vi "Read Video.vi"(8 "error in (no error)":errorcluster, 11 "input cluster":T4={"Video Resolution"=enum."FREENECT_RESOLUTION_LOW", "Video Format"=enum."FREENECT_VIDEO_RGB", "Depth Format"=enum."FREENECT_DEPTH_11BIT", "Depth Resolution"=enum."FREENECT_RESOLUTION_LOW"}) -> (0 "error out":errorcluster, 1 "raw data":u16[](array[numeric]), 3 "RGB image":picture)   [LabVIEW 2015]
uses:
  Video Resolution Control.ctl
  Video Format Control.ctl
  Depth Resolution Control.ctl
  <vilib>/picture/picture.llb/Draw True-Color Pixmap.vi
  libkinect_wrapper.dll
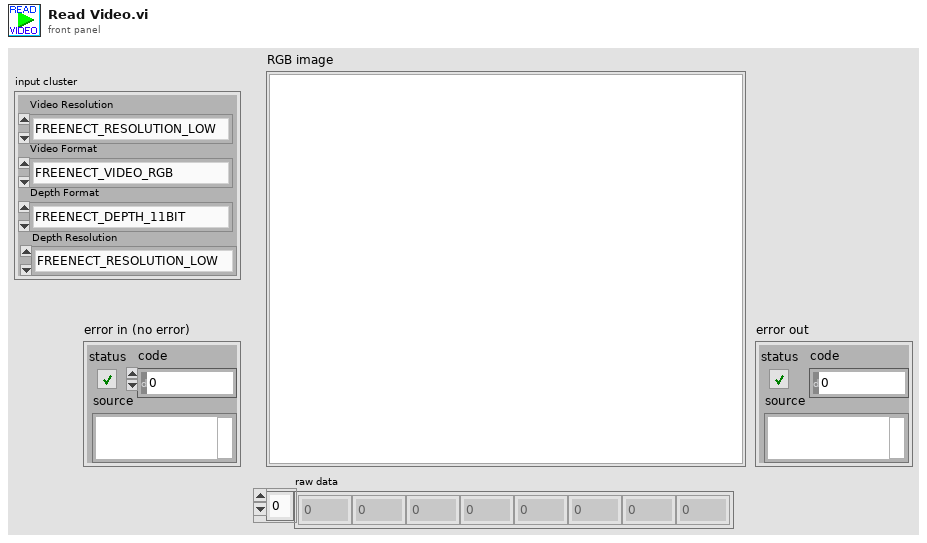
[diagram p1: front panel]
types:
  T1 = typedef "Video Resolution Control.ctl" = enum32{"FREENECT_RESOLUTION_LOW", "FREENECT_RESOLUTION_MEDIUM", "FREENECT_RESOLUTION_HIGH"}
  T2 = typedef "Video Format Control.ctl" = enum32{"FREENECT_VIDEO_RGB", "FREENECT_VIDEO_BAYER", "FREENECT_VIDEO_IR_8BIT", "FREENECT_VIDEO_IR_10BIT", "FREENECT_VIDEO_IR_10BIT_PACKED", "FREENECT_VIDEO_YUV_RGB", "FREENECT_VIDEO_YUV_RAW"}
  T3 = typedef "Depth Resolution Control.ctl" = enum16{"FREENECT_RESOLUTION_TINY", "FREENECT_RESOLUTION_LOW", "FREENECT_RESOLUTION_MEDIUM"}
  T4 = cluster{"Video Resolution":T1, "Video Format":T2, "Depth Format":enum32{"FREENECT_DEPTH_11BIT", "FREENECT_DEPTH_10BIT", "FREENECT_DEPTH_11BIT_PACKED", "FREENECT_DEPTH_10BIT_PACKED", "FREENECT_DEPTH_REGISTERED", "FREENECT_DEPTH_MM"}, "Depth Resolution":T3}
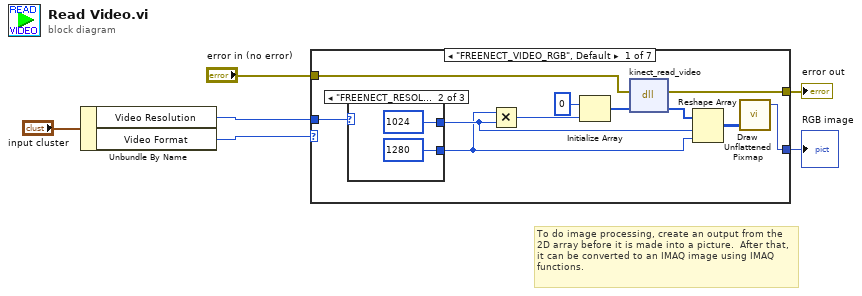
[diagram p0: block diagram]
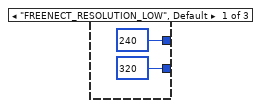
[diagram p2: hidden frame]
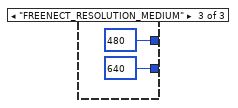
[diagram p3: hidden frame]
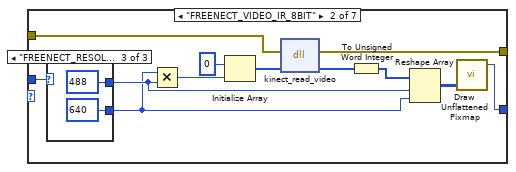
[diagram p4: hidden frame]
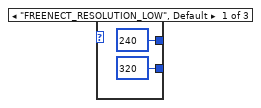
[diagram p5: hidden frame]
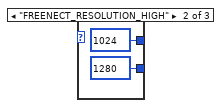
[diagram p6: hidden frame]
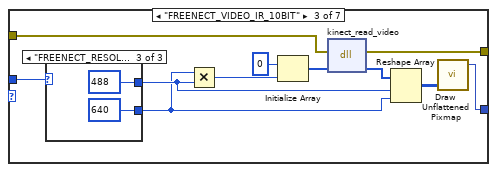
[diagram p7: hidden frame]
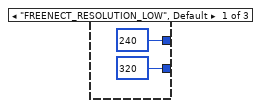
[diagram p8: hidden frame]
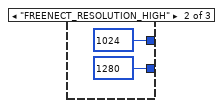
[diagram p9: hidden frame]
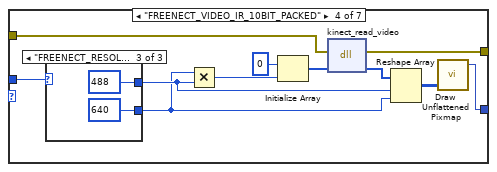
[diagram p10: hidden frame]
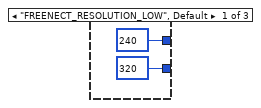
[diagram p11: hidden frame]
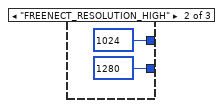
[diagram p12: hidden frame]
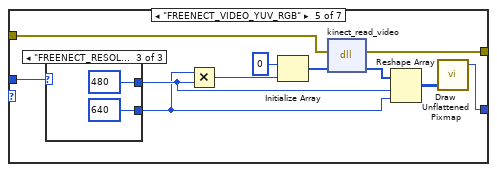
[diagram p13: hidden frame]
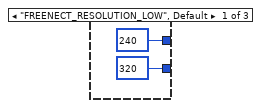
[diagram p14: hidden frame]
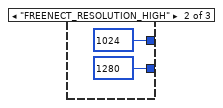
[diagram p15: hidden frame]
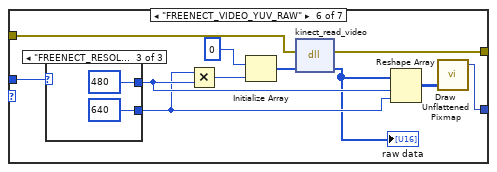
[diagram p16: hidden frame]
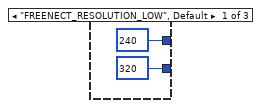
[diagram p17: hidden frame]
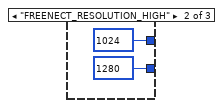
[diagram p18: hidden frame]
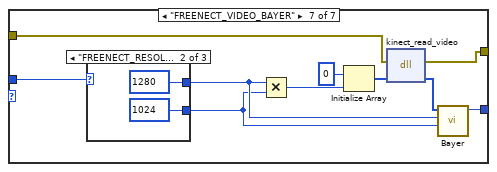
[diagram p19: hidden frame]
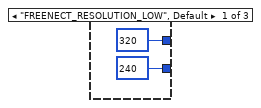
[diagram p20: hidden frame]
diagram:
  # "To do image processing, create an output from the 2D array before it is made into a picture.  After that, it can be converted to an IMAQ image using IMAQ functions."
  n1 = Unbundle By Name("input cluster") -> ("Video Resolution"=w4:T1, "Video Format"=w5:T2)
  n2 = case shown="\"FREENECT_VIDEO_RGB\", Default" w5 {
    tunnel: w4 -> [w17 w27 w42 w61 w86 w103 w112]
    tunnel: [w11 w29 w44 w63 w80 w94 w113] -> w3
    tunnel: "error in (no error)" -> [w10 w28 w43 w62 w79 w99 w115]
    tunnel: [w9 w30 w45 w64 w78 w98 w114] -> w1
    frame "FREENECT_VIDEO_RGB", Default {
      n3 = case shown="\"FREENECT_RESOLUTION_HIGH\"" w17 {
        tunnel: [240 1024 480] -> w8
        tunnel: [320 1280 640] -> w7
        frame "FREENECT_RESOLUTION_LOW", Default {
        }
        frame "FREENECT_RESOLUTION_HIGH" {
        }
        frame "FREENECT_RESOLUTION_MEDIUM" {
        }
      }
      n4 = Multiply(x=w7, y=w8) -> (x*y=w16:i32)
      n5 = Initialize Array(u32 0 ("U32"), w16) -> (w15:u32[])
      n6 = dll-call lib="libkinect_wrapper.*" fn="kinect_read_video"(error in=w10, "video"=w15) -> (error out=w9:errorcluster, "video"=w13:u32[])  [unwired: 3 in, 1 out]
      n7 = Reshape Array(w13, w8, w7) -> (w12:u32[][])
      n8 = call-poly <vilib>:"Draw Unflattened Pixmap.vi"("data (RGB format)"=w12) -> ("new picture"=w11:picture)  [unwired: 8 in]
    }
    frame "FREENECT_VIDEO_IR_8BIT" {
      n9 = case shown="\"FREENECT_RESOLUTION_MEDIUM\"" w27 {
        tunnel: [240 1024 488] -> w32
        tunnel: [320 1280 640] -> w31
        frame "FREENECT_RESOLUTION_LOW", Default {
        }
        frame "FREENECT_RESOLUTION_HIGH" {
        }
        frame "FREENECT_RESOLUTION_MEDIUM" {
        }
      }
      n10 = Multiply(x=w31, y=w32) -> (x*y=w35:i32)
      n11 = Initialize Array(u8 0 ("U32"), w35) -> (w34:u8[])
      n12 = dll-call lib="libkinect_wrapper.*" fn="kinect_read_video"(error in=w28, "video"=w34) -> (error out=w30:errorcluster, "video"=w26:u8[])  [unwired: 3 in, 1 out]
      n13 = To Unsigned Word Integer(number=w26) -> (unsigned 16bit integer=w25:u16[])
      n14 = Reshape Array(w25, w32, w31) -> (w24:u16[][])
      n15 = call-poly <vilib>:"Draw Unflattened Pixmap.vi"("data (RGB format)"=w24) -> ("new picture"=w29:picture)  [unwired: 8 in]
    }
    frame "FREENECT_VIDEO_IR_10BIT" {
      n16 = case shown="\"FREENECT_RESOLUTION_MEDIUM\"" w42 {
        tunnel: [240 1024 488] -> w47
        tunnel: [320 1280 640] -> w46
        frame "FREENECT_RESOLUTION_LOW", Default {
        }
        frame "FREENECT_RESOLUTION_HIGH" {
        }
        frame "FREENECT_RESOLUTION_MEDIUM" {
        }
      }
      n17 = Multiply(x=w46, y=w47) -> (x*y=w52:i32)
      n18 = Initialize Array(u16 0 ("U32"), w52) -> (w51:u16[])
      n19 = dll-call lib="libkinect_wrapper.*" fn="kinect_read_video"(error in=w43, "video"=w51) -> (error out=w45:errorcluster, "video"=w49:u16[])  [unwired: 3 in, 1 out]
      n20 = Reshape Array(w49, w47, w46) -> (w48:u16[][])
      n21 = call-poly <vilib>:"Draw Unflattened Pixmap.vi"("data (RGB format)"=w48) -> ("new picture"=w44:picture)  [unwired: 8 in]
    }
    frame "FREENECT_VIDEO_IR_10BIT_PACKED" {
      n22 = case shown="\"FREENECT_RESOLUTION_MEDIUM\"" w61 {
        tunnel: [240 1024 488] -> w66
        tunnel: [320 1280 640] -> w65
        frame "FREENECT_RESOLUTION_LOW", Default {
        }
        frame "FREENECT_RESOLUTION_HIGH" {
        }
        frame "FREENECT_RESOLUTION_MEDIUM" {
        }
      }
      n23 = Multiply(x=w65, y=w66) -> (x*y=w69:i32)
      n24 = Initialize Array(u16 0 ("U32"), w69) -> (w68:u16[])
      n25 = dll-call lib="libkinect_wrapper.*" fn="kinect_read_video"(error in=w62, "video"=w68) -> (error out=w64:errorcluster, "video"=w60:u16[])  [unwired: 3 in, 1 out]
      n26 = Reshape Array(w60, w66, w65) -> (w59:u16[][])
      n27 = call-poly <vilib>:"Draw Unflattened Pixmap.vi"("data (RGB format)"=w59) -> ("new picture"=w63:picture)  [unwired: 8 in]
    }
    frame "FREENECT_VIDEO_YUV_RGB" {
      n28 = case shown="\"FREENECT_RESOLUTION_MEDIUM\"" w86 {
        tunnel: [240 1024 480] -> w77
        tunnel: [320 1280 640] -> w76
        frame "FREENECT_RESOLUTION_LOW", Default {
        }
        frame "FREENECT_RESOLUTION_HIGH" {
        }
        frame "FREENECT_RESOLUTION_MEDIUM" {
        }
      }
      n29 = Multiply(x=w76, y=w77) -> (x*y=w85:i32)
      n30 = Initialize Array(u32 0 ("U32"), w85) -> (w84:u32[])
      n31 = dll-call lib="libkinect_wrapper.*" fn="kinect_read_video"(error in=w79, "video"=w84) -> (error out=w78:errorcluster, "video"=w82:u32[])  [unwired: 3 in, 1 out]
      n32 = Reshape Array(w82, w77, w76) -> (w81:u32[][])
      n33 = call-poly <vilib>:"Draw Unflattened Pixmap.vi"("data (RGB format)"=w81) -> ("new picture"=w80:picture)  [unwired: 8 in]
    }
    frame "FREENECT_VIDEO_YUV_RAW" {
      n34 = case shown="\"FREENECT_RESOLUTION_MEDIUM\"" w103 {
        tunnel: [240 1024 480] -> w97
        tunnel: [320 1280 640] -> w96
        frame "FREENECT_RESOLUTION_LOW", Default {
        }
        frame "FREENECT_RESOLUTION_HIGH" {
        }
        frame "FREENECT_RESOLUTION_MEDIUM" {
        }
      }
      n35 = Multiply(x=w96, y=w97) -> (x*y=w102:i32)
      n36 = Initialize Array(u16 0 ("U32"), w102) -> (w101:u16[])
      n37 = dll-call lib="libkinect_wrapper.*" fn="kinect_read_video"(error in=w99, "video"=w101) -> (error out=w98:errorcluster, "video"=w95:u16[])  [unwired: 3 in, 1 out]
      "raw data" <- w95
      n38 = Reshape Array(w95, w97, w96) -> (w93:u16[][])
      n39 = call-poly <vilib>:"Draw Unflattened Pixmap.vi"("data (RGB format)"=w93) -> ("new picture"=w94:picture)  [unwired: 8 in]
    }
    frame "FREENECT_VIDEO_BAYER" {
      n40 = case shown="\"FREENECT_RESOLUTION_HIGH\"" w112 {
        tunnel: [320 1280 640] -> w111
        tunnel: [240 1024 480] -> w110
        frame "FREENECT_RESOLUTION_LOW", Default {
        }
        frame "FREENECT_RESOLUTION_HIGH" {
        }
        frame "FREENECT_RESOLUTION_MEDIUM" {
        }
      }
      n41 = Multiply(x=w111, y=w110) -> (x*y=w119:i32)
      n42 = Initialize Array(u8 0, w119) -> (w118:u8[])
      n43 = dll-call lib="libkinect_wrapper.*" fn="kinect_read_video"(error in=w115, "video"=w118) -> (error out=w114:errorcluster, "video"=w117:u8[])  [unwired: 3 in, 1 out]
      n44 = call "Bayer.vi"("Height"=w110, "Width"=w111, "Array"=w117) -> ("new picture"=w113:picture)  [unwired: 8 in]
    }
  }
  "error out" <- w1
  "RGB image" <- w3
